vi "Panel.vi"(11 "Team Config Panel in":refnum<class "Team Config Panel.lvclass">) -> ()   [LabVIEW 2020, in "SB App.lvlib" / "Team Config Panel.lvclass"]
uses:
  Team Config Panel.lvclass
  C:/Program Files (x86)/National Instruments/LabVIEW 2020/vi.lib/IlluminatedG/IG OOPanel/OOPanel/Panel/Panel.lvclass
  <vilib>/IlluminatedG/IG OOPanel/OOPanel/Panel/Basic UI State.ctl
  Update Team Data.ctl
  SquareBattle/Team/Team.lvclass
  Team Config Panel.lvclass/Team Config Panel.ctl
  SquareBattle/Team/Team.lvclass/Team.ctl
  <vilib>/IlluminatedG/IG OOPanel/OOPanel/Panel/Panel.lvclass
  <vilib>/IlluminatedG/IG OOPanel/OOPanel/OOPanel.lvlib
  SquareBattle/SquareBattle.lvlib
panel:
  out "Player":string
  out "Team Name":string
  in  "Remove":bool
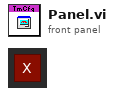
[diagram p1: front panel]
types:
  T1 = typedef "OOPanel.lvlib/Panel.lvclass/Basic UI State.ctl" = enum16{"Init", "Run", "Close"}
  T2 = typedef "SB App.lvlib/Team Config Panel.lvclass/Update Team Data.ctl" = cluster{"Team":refnum<class "Team.lvclass">}
  T3 = typedef "SB App.lvlib/Team Config Panel.lvclass/Incoming Events.ctl" = cluster{"Team Index":refnum<user-event>, "Position Enabled":refnum<user-event>, "Update Team":refnum<user-event>, "Start Position":refnum<user-event>}
  T4 = typedef "OOPanel.lvlib/Panel.lvclass/Panel Events.ctl" = cluster{"Visbility":refnum<user-event>, "Close":refnum<user-event>}
  T5 = typedef "SquareBattle.lvlib/Team ID.ctl" = u32
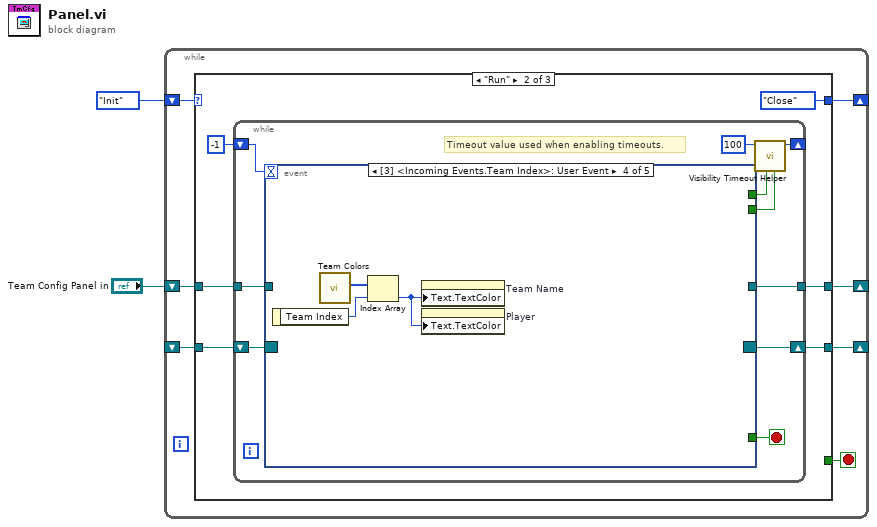
[diagram p0: block diagram]
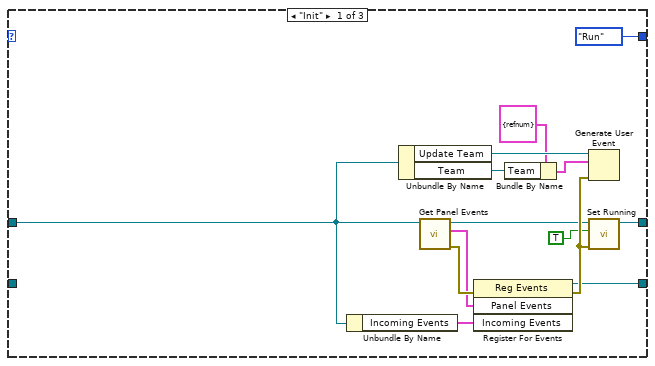
[diagram p2: hidden frame]
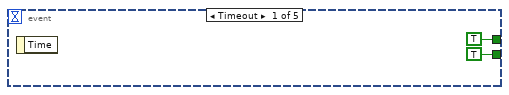
[diagram p3: hidden frame]
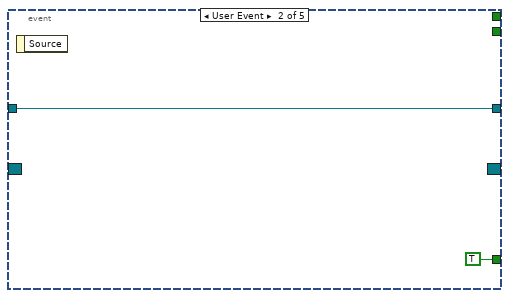
[diagram p4: hidden frame]
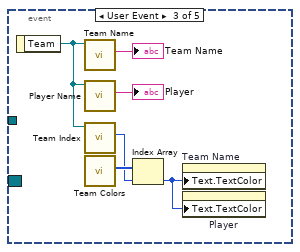
[diagram p5: hidden frame]
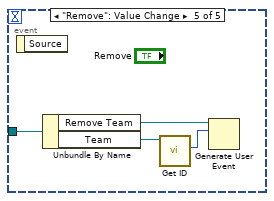
[diagram p6: hidden frame]
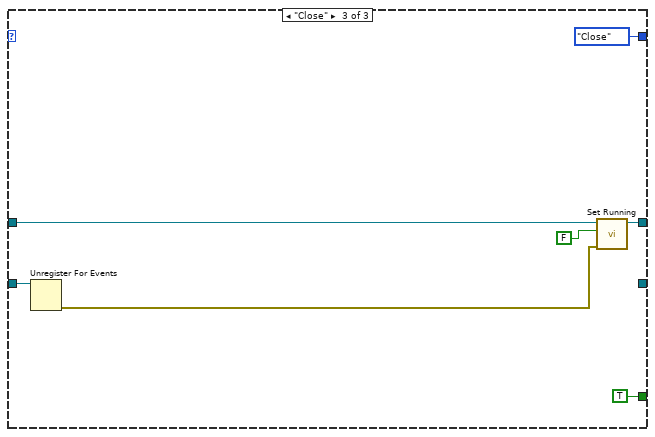
[diagram p7: hidden frame]
diagram:
  n1 = while {
    shift-right: [w8] -> _
    shift-left: _ -> [w9]
    shift-right: [w6] -> _
    shift-left: Basic_UI_State."Init" ("Basic UI State") -> [w7]
    shift-right: [w4] -> _
    shift-left: "Team Config Panel in" -> [w3]
    stop <- w5 stop-if-true
    n2 = case shown="\"Run\"" w7 {
      tunnel: w9 -> [_ w29 w59]
      tunnel: [w17 w27 _] -> w8
      tunnel: [Basic_UI_State."Run" ("Basic UI State") Basic_UI_State."Close" ("Basic UI State") Basic_UI_State."Close" ("Basic UI State")] -> w6
      tunnel: [_ _ TRUE] -> w5
      tunnel: [w16 w24 w57] -> w4
      tunnel: w3 -> [w14 w25 w58]
      frame "Init" {
        n3 = Unbundle By Name(w14) -> ("Incoming Events"=w15:T3)
        n4 = Unbundle By Name(w14) -> ("Update Team"=w13:refnum<user-event>, "Team"=w10:refnum<class "Team.lvclass">)
        n5 = call <vilib>:"Get Panel Events.vi"("Panel in"=w14) -> ("error out"=w22:errorcluster, "Panel Events"=w19:T4, "Panel out"=w20:refnum<class "Team Config Panel.lvclass">)  [unwired: 8 in]
        n6 = register-events(error in=w22, w19, w15) -> (reference out=w17:refnum<event-registration>, error out=w23:errorcluster)  [unwired: 1 in]
        n7 = Bundle By Name(cluster=T2 {"Team"=refnum} ("event data"), "Team"=w10) -> (w11:T2)
        n8 = Generate User Event(user event=w13, event data cluster=w11, error in=w23) -> ()  [unwired: 1 in, 2 out]
        n9 = call <vilib>:"Set Running.vi"("error in (no error)"=w23, "Running"=TRUE, "Panel in"=w20) -> ("Panel out"=w16:refnum<class "Team Config Panel.lvclass">)  [unwired: 7 in, 1 out]
      }
      frame "Run" {
        n10 = while {
          shift-right: [w35] -> w27
          shift-left: w29 -> [w36]
          shift-right: [w38] -> _
          shift-left: -1 ("Timeout") -> [w37]
          tunnel: w25 -> [w31]
          tunnel: [w30] -> w24
          stop <- w32 stop-if-true
          # "Timeout value used when enabling timeouts."
          n11 = event shown="[3] <Incoming Events.Team Index>: User Event" {
            selector: w36 -> [_ _ _ _ _]
            dyn-events: [_ _ _ _ _] -> w35
            timeout: w37 -> [_ _ _ _ _]
            tunnel: [TRUE _ _ _ _] -> w34
            tunnel: [TRUE _ _ _ _] -> w33
            tunnel: [_ TRUE _ _ _] -> w32
            tunnel: w31 -> [_ w42 _ _ w55]
            tunnel: [_ w42 _ _ _] -> w30
            event Timeout {
              n12 = event-data() -> ()  [unwired: 1 in, 1 out]
            }
            event User Event {
              n13 = event-data() -> ()  [unwired: 1 in, 1 out]
            }
            event User Event {
              n14 = event-data() -> ("Team"=w46:refnum<class "Team.lvclass">)  [unwired: 1 in]
              n15 = call-dynamic "Team Name.vi"("Team in"=w46) -> ("Team Name"=→"Team Name":string)  [unwired: 10 in]
              n16 = call-dynamic "Player Name.vi"("Team"=w46) -> ("Player Name"=→"Player":string)  [unwired: 10 in]
              n17 = call "Team Index.vi"("Team"=w46) -> ("Team Index"=w48:i32)  [unwired: 10 in]
              n18 = call "Team Colors.vi"() -> ("Team Colors"=w49:u32[])  [unwired: 11 in]
              n19 = Index Array(array=w49, index=w48) -> (element=w47:u32)
              n20 = property on="Team Name" class="Str"("Text.TextColor"=w47) -> ()  [unwired: 2 in, 2 out]
              n21 = property on="Player" class="Str"("Text.TextColor"=w47) -> ()  [unwired: 2 in, 2 out]
            }
            event User Event {
              n22 = event-data() -> ("Team Index"=w51:i32)  [unwired: 1 in]
              n23 = call "Team Colors.vi"() -> ("Team Colors"=w52:u32[])  [unwired: 11 in]
              n24 = Index Array(array=w52, index=w51) -> (element=w50:u32)
              n25 = property on="Team Name" class="Str"("Text.TextColor"=w50) -> ()  [unwired: 2 in, 2 out]
              n26 = property on="Player" class="Str"("Text.TextColor"=w50) -> ()  [unwired: 2 in, 2 out]
            }
            event "Remove": Value Change {
              n27 = event-data() -> ()  [unwired: 1 in, 1 out]
              n28 = Unbundle By Name(w55) -> ("Remove Team"=w56:refnum<user-event>, "Team"=w54:refnum<class "Team.lvclass">)
              n29 = call "Get ID.vi"("Team in"=w54) -> ("Team ID"=w53:T5)  [unwired: 10 in]
              n30 = Generate User Event(user event=w56, event data cluster=w53) -> ()  [unwired: 2 in, 2 out]
            }
          }
          n31 = call <vilib>:"Visibility Timeout Helper.vi"("Update?"=w33, "Use Timeout?"=w34, "Visible Timeout mS"=100) -> ("Timeout"=w38:i32)  [unwired: 8 in]
        }
      }
      frame "Close" {
        n32 = Unregister For Events(event registration refnum=w59) -> (error out=w61:errorcluster)  [unwired: 1 in]
        n33 = call <vilib>:"Set Running.vi"("error in (no error)"=w61, "Running"=FALSE, "Panel in"=w58) -> ("Panel out"=w57:refnum<class "Team Config Panel.lvclass">)  [unwired: 7 in, 1 out]
      }
    }
  }
